vi "Timer 2.vi"(8 "error in (no error)":errorcluster, 9 "Message":T1, 11 "Timer":refnum<queue>) -> (0 "error out":errorcluster, 2 "Elapsed Time (ms)":string)   [LabVIEW 2014]
uses:
  Engine/Message.ctl
  support/Message Queue/Message Cluster.ctl
  Teszt/Teszt.ctl
  Teszt/Command.ctl
  support/Message Queue/Enqueue Message (Single).vi
  support/Message Queue/Message Queue.lvlib
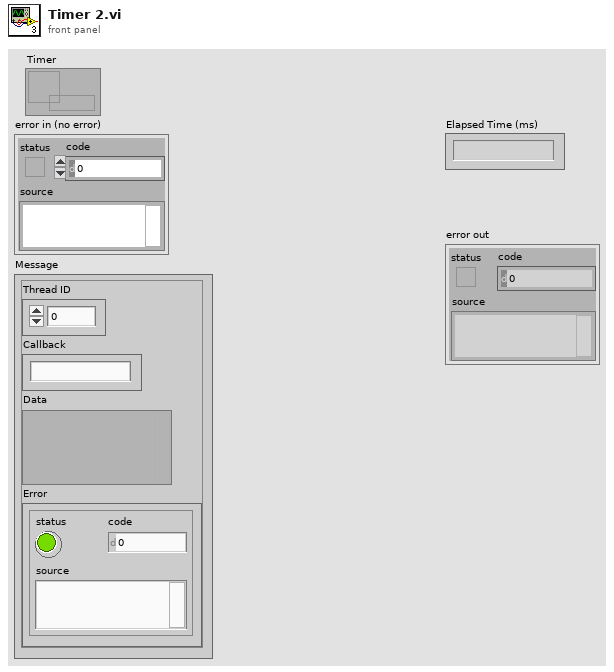
[diagram p1: front panel]
types:
  T1 = typedef "Message.ctl" = cluster{"Thread ID":u16, "Callback":string, "Data":variant, "Error":errorcluster}
  T2 = typedef "Teszt.ctl" = cluster{"Thread ID":dbl, "Mérésszám":string, "Mérés/Utasítás":string, "Command":T3, "Min":string, "Max":string, "Aktív?":bool, "Log?":bool, "Kiértékelés":bool, "Etalon 1 exp":bool, "Etalon 2 exp":bool, "Etalon 3 exp":bool, "Etalon 4 exp":bool, "Etalon 5 exp":bool}
  T3 = typedef "Command.ctl" = cluster{"Parancs":string, "Paraméter 1":string, "Paraméter 2":string, "Paraméter 3":string, "Paraméter 4":string, "Paraméter 5":string, "Eredmény":string}
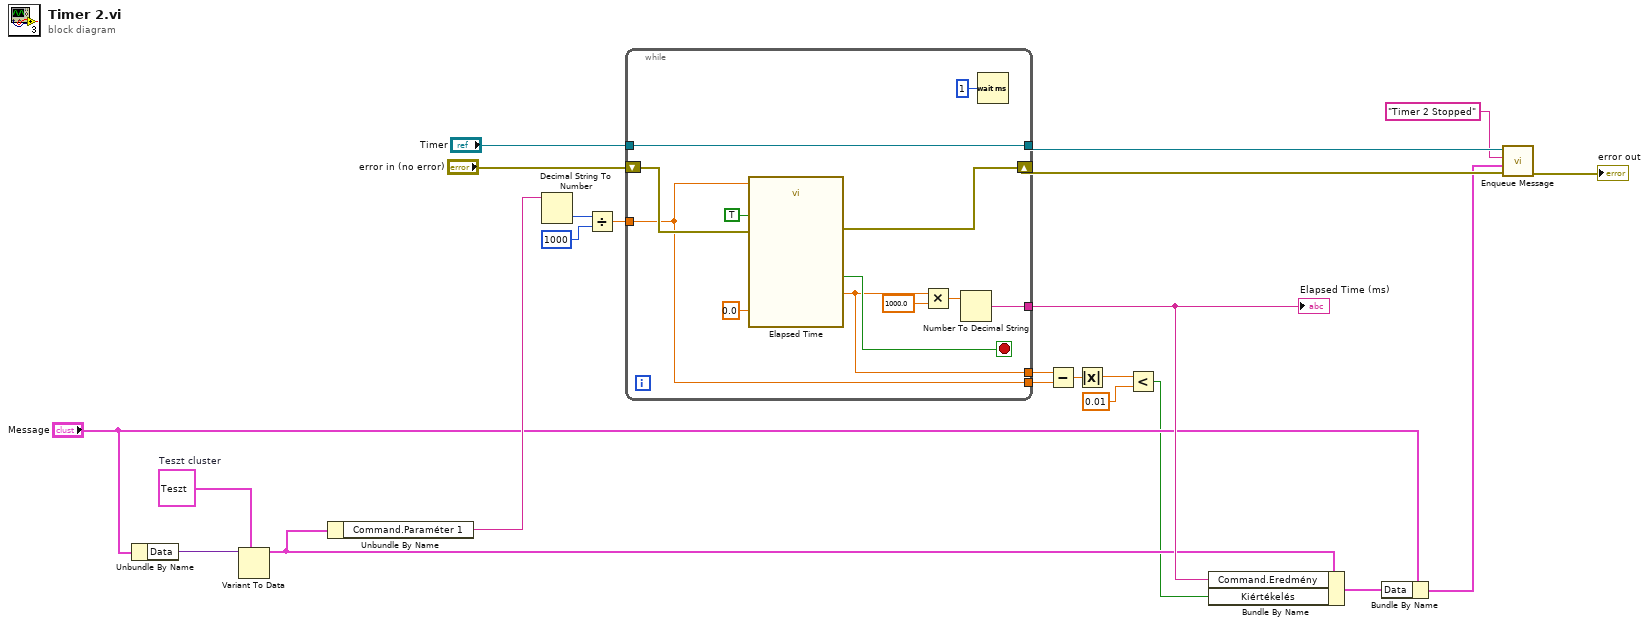
[diagram p0: block diagram]
diagram:
  w15 = T2 {"Thread ID"=0.0, "Mérésszám"="", "Mérés/Utasítás"="", "Command"={"Parancs"="", "Paraméter 1"="", "Paraméter 2"="", "Paraméter 3"="", "Paraméter 4"="", "Paraméter 5"="", "Eredmény"=""}, "Min"="", "Max"="", "Aktív?"=FALSE, "Log?"=FALSE, "Kiértékelés"=FALSE, "Etalon 1 exp"=FALSE, "Etalon 2 exp"=FALSE, "Etalon 3 exp"=FALSE, "Etalon 4 exp"=FALSE, "Etalon 5 exp"=FALSE}  # Teszt cluster
  n1 = Unbundle By Name("Message") -> ("Data"=w14:variant)
  n2 = Variant To Data(type=w15, Variant=w14) -> (data=w12:T2)  [unwired: 1 in, 1 out]
  n3 = Unbundle By Name(w12) -> ("Command.Paraméter 1"=w11:string)
  n4 = Decimal String To Number(string=w11) -> (number=w23:i32)  [unwired: 2 in, 1 out]
  n5 = Divide(x=w23, y=1000) -> (x/y=w21:dbl)
  n6 = while {
    tunnel: [w35] -> w18
    tunnel: "Timer" -> [w35]
    tunnel: [w30] -> w13
    tunnel: w21 -> [w27]
    shift-right: [w28] -> w19
    shift-left: "error in (no error)" -> [w29]
    tunnel: [w27] -> w9
    tunnel: [w26] -> w8
    stop <- w33 stop-if-true
    n7 = call "Elapsed Time"("Time Target (s)"=w27, "Auto Reset"=TRUE, "error in (no error)"=w29, "Set Start Time (s)"=0.0) -> ("Elapsed Time (s)"=w26:dbl, "Time has Elapsed"=w33:bool, "error out"=w28:errorcluster)  [unwired: 8 in, 5 out]
    n8 = Multiply(x=w26, y=1000.0) -> (x*y=w31:dbl)
    n9 = Number To Decimal String(number=w31) -> (decimal integer string=w30:string)  [unwired: 1 in]
    n10 = Wait (ms)(milliseconds to wait=u32 1) -> ()  [unwired: 1 out]
  }
  "Elapsed Time (ms)" <- w13
  n11 = Subtract(x=w8, y=w9) -> (x-y=w7:dbl)
  n12 = Absolute Value(x=w7) -> (abs(x)=w6:dbl)
  n13 = Less?(x=w6, y=0.01) -> (x < y?=w4:bool)
  n14 = Bundle By Name(cluster=w12, "Command.Eredmény"=w13, "Kiértékelés"=w4) -> (w3:T2)
  n15 = Bundle By Name(cluster="Message", "Data"=w3) -> (w2:T1)
  n16 = call-poly "Enqueue Message.vi"("error in (no error)"=w19, "Message Data"=w2, "Message"="Timer 2 Stopped", "Message Queue"=w18) -> ("error out"=→"error out":errorcluster)  [unwired: 6 in, 1 out]
